vi "Initialise.vi"(8 "error in (no error)":errorcluster, 10 "Message in":refnum<class "InitialiseMessage.lvclass">, 11 "Piezo in":refnum<class "Piezo.lvclass">) -> (0 "error out":errorcluster, 3 "Piezo out":refnum<class "Piezo.lvclass">)   [LabVIEW 2012, in "Piezo.lvclass"]
doc: "This method is called when an initialise message is received. It mainly initialises the RabbitMQ connectivity. \n\nOverride this method when your component needs special initialisation (e.g. of software or hardware resources). In that case, don't forget to call the parent for proper implementation. If your component owns subcomponents, they count as resources, so you have to initialise them by calling their own initialise functions"
uses:
  Piezo.lvclass
  <vilib>/Distrio/Murmex/InitialiseMessage/InitialiseMessage.lvclass
  <vilib>/Distrio/Murmex/Murmex/Murmex.lvclass
  Piezo.lvclass/Piezo.ctl
  <vilib>/DAQmx/create/channels.llb/DAQmx Create Channel (AO-Voltage-Basic).vi
panel:
  # "This method is called when the INTIALISE\ntrigger is sent. \n\nOverride this method when your component needs to\nrespond to this trigger. \n\nCall parent for proper implementation"
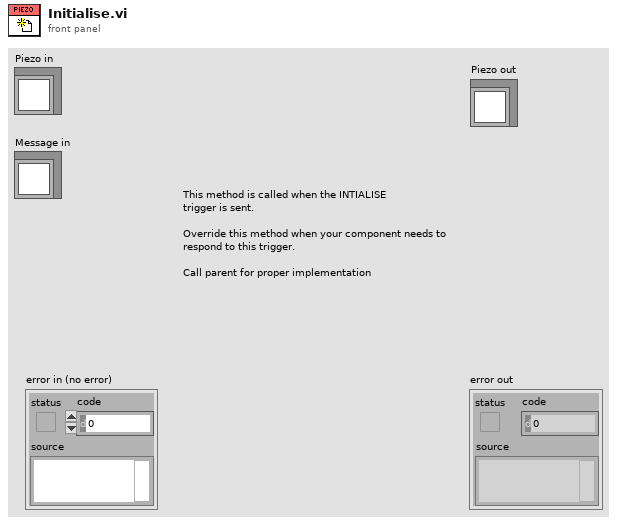
[diagram p1: front panel]
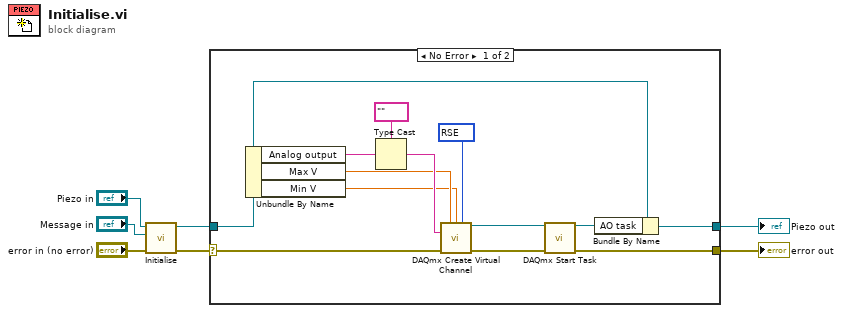
[diagram p0: block diagram]
diagram:
  n1 = call-parent "Initialise.vi"("error in (no error)"="error in (no error)", "Message in"="Message in", "Murmex in"="Piezo in") -> ("error out"=w4:errorcluster, "Murmex out"=w1:refnum<class "Piezo.lvclass">)  [unwired: 7 in]
  n2 = case shown="No Error" w4 {
    selector: w4 -> [w20 w22]
    tunnel: [w11 w22] -> w3
    tunnel: [w13 w21] -> w2
    tunnel: w1 -> [w14 w21]
    frame No Error {
      w8 = 10083 items=["Default"=-1, "RSE"=10083, "Differential"=10106, "Pseudodifferential"=12529] ("output terminal configuration")
      n3 = Unbundle By Name(w14) -> ("Analog output"=w19:string, "Max V"=w16:dbl, "Min V"=w15:dbl)
      n4 = Type Cast(type=tag "" ("physical channels"), x=w19) -> (*(type *) &x=w17:tag)
      n5 = call-poly <vilib>:"DAQmx Create Virtual Channel.vi"("maximum value"=w16, "minimum value"=w15, "output terminal configuration"=w8, "physical channels"=w17, "error in"=w20) -> ("task out"=w10:refnum<k21>, "error out"=w12:errorcluster)  [unwired: 9 in]
      n6 = call <vilib>:"DAQmx Start Task.vi"("task/channels in"=w10, "error in"=w12) -> ("task out"=w9:refnum<k21>, "error out"=w11:errorcluster)  [unwired: 12 in]
      n7 = Bundle By Name(cluster=w14, "AO task"=w9) -> (w13:refnum<class "Piezo.lvclass">)
    }
    frame Error {
    }
  }
  "error out" <- w3
  "Piezo out" <- w2
